vi "Initialise.vi"(8 "error in (no error)":errorcluster, 10 "Message in":refnum<class "InitialiseMessage.lvclass">, 11 "StageSPIM in":refnum<class "StageSPIM.lvclass">) -> (0 "error out":errorcluster, 3 "StageSPIM out":refnum<class "StageSPIM.lvclass">)   [LabVIEW 2012, in "StageSPIM.lvclass"]
doc: "This method is called when an initialise message is received. It mainly initialises the RabbitMQ connectivity. \n\nOverride this method when your component needs special initialisation (e.g. of software or hardware resources). In that case, don't forget to call the parent for proper implementation. If your component owns subcomponents, they count as resources, so you have to initialise them by calling their own initialise functions"
uses:
  StageSPIM.lvclass
  <vilib>/Distrio/Murmex/InitialiseMessage/InitialiseMessage.lvclass
  <vilib>/Distrio/Murmex/Murmex/Murmex.lvclass
  StageSPIM.lvclass/StageSPIM.ctl
panel:
  # "This method is called when the INTIALISE\ntrigger is sent. \n\nOverride this method when your component needs to\nrespond to this trigger. \n\nCall parent for proper implementation"
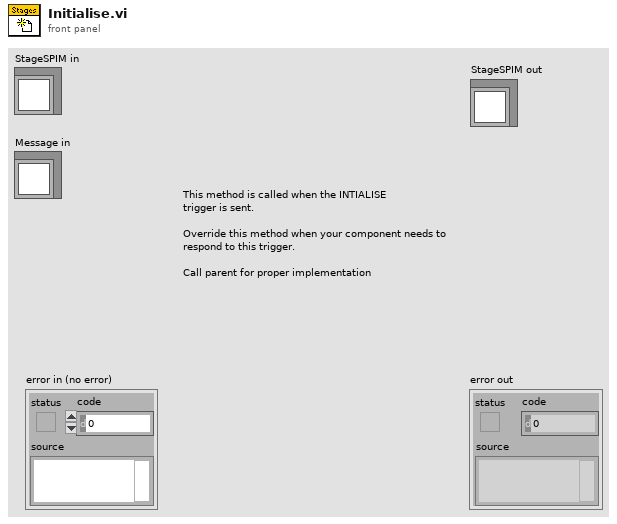
[diagram p1: front panel]
types:
  T1 = cluster{"Register DC":bool, "DaisyChain Search?":bool, "Device ID":i32}[][]
  T2 = cluster{"RON Affected axes":string[], "Reference mode":bool[], "Check FRF?":bool}
  T3 = typedef "StageSPIM.lvclass/port_control.ctl" = i32
  T4 = typedef "StageSPIM.lvclass/baud_rate_control.ctl" = u16
  T5 = typedef "StageSPIM.lvclass/connection_type.ctl" = enum16{"RS232", "RS232 DaisyChain", "USB", "USB_DaisyChain"}
  T6 = cluster{"Register DC":bool, "DaisyChain Search?":bool, "Device ID":i32}
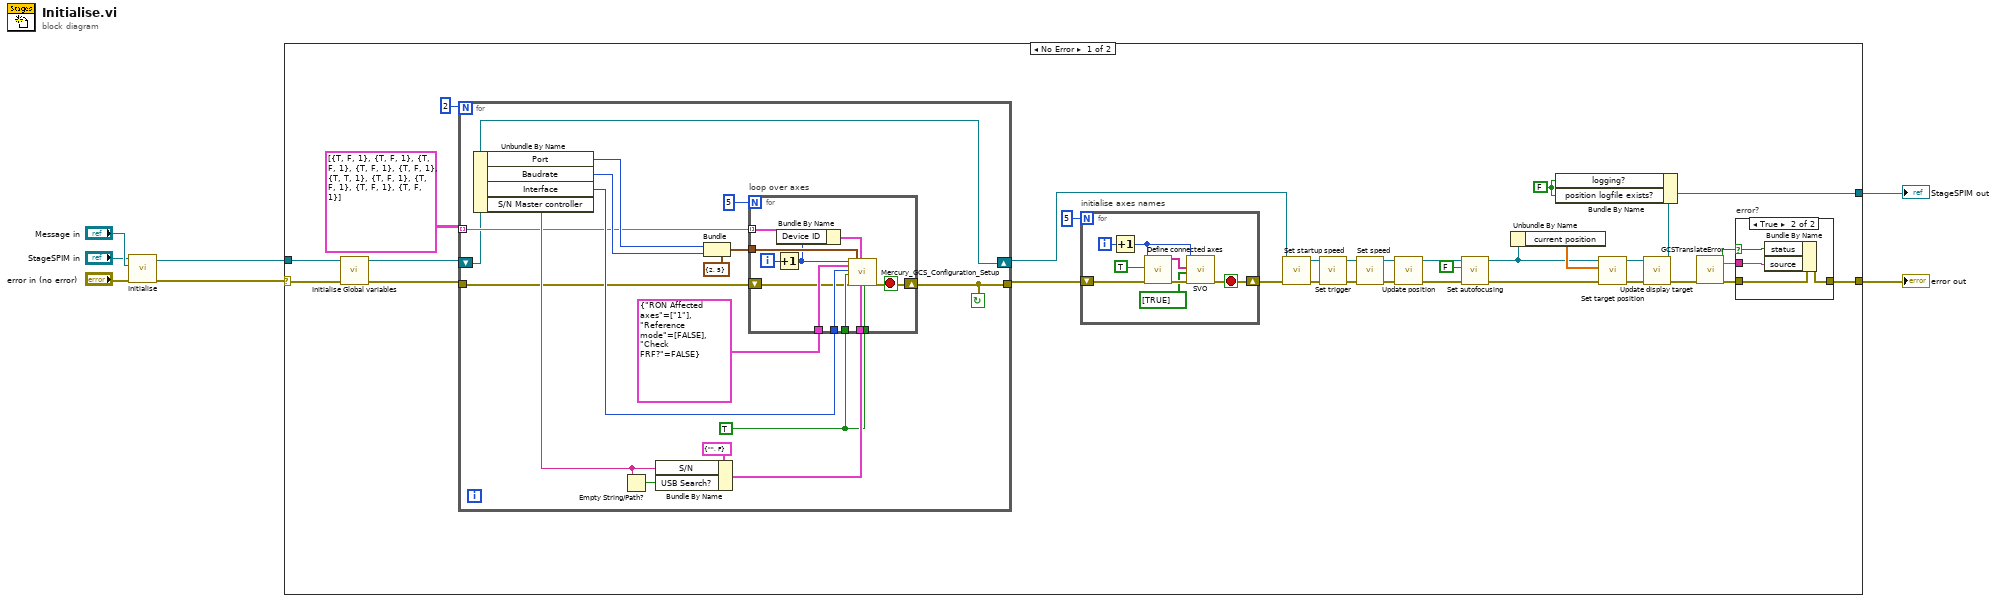
[diagram p0: block diagram]
diagram:
  n1 = call-parent "Initialise.vi"("error in (no error)"="error in (no error)", "Message in"="Message in", "Murmex in"="StageSPIM in") -> ("error out"=w4:errorcluster, "Murmex out"=w3:refnum<class "StageSPIM.lvclass">)  [unwired: 7 in]
  n2 = case shown="No Error" w4 {
    selector: w4 -> [w30 w82]
    tunnel: w3 -> [w28 w81]
    tunnel: [w9 w81] -> w2
    tunnel: [w31 w82] -> w1
    frame No Error {
      w8 = FALSE ("settings.logging?")
      n3 = call-dynamic "Initialise Global variables.vi"("error in (no error)"=w30, "StageSPIM in"=w28) -> ("error out"=w29:errorcluster, "StageSPIM out"=w27:refnum<class "StageSPIM.lvclass">)  [unwired: 8 in]
      n4 = for {
        N: 2 -> [_]
        tunnel: [w41] -> w34
        tunnel: w29 -> [w44]
        tunnel: T1 [[{"Register DC"=TRUE, "DaisyChain Search?"=FALSE, "Device ID"=1}, {"Register DC"=TRUE, "DaisyChain Search?"=FALSE, "Device ID"=1}, {"Register DC"=TRUE, "DaisyChain Search?"=FALSE, "Device ID"=1}, {"Register DC"=TRUE, "DaisyChain Search?"=FALSE, "Device ID"=1}, {"Register DC"=TRUE, "DaisyChain Search?"=FALSE, "Device ID"=1}], [{"Register DC"=TRUE, "DaisyChain Search?"=TRUE, "Device ID"=1}, {"Register DC"=TRUE, "DaisyChain Search?"=FALSE, "Device ID"=1}, {"Register DC"=TRUE, "DaisyChain Search?"=FALSE, "Device ID"=1}, {"Register DC"=TRUE, "DaisyChain Search?"=FALSE, "Device ID"=1}, {"Register DC"=TRUE, "DaisyChain Search?"=FALSE, "Device ID"=1}]] -> [w43] mode=indexing
        shift-right: [w42] -> w17
        shift-left: w27 -> [w42]
        stop <- w41 continue-if-true
        w49 = TRUE ("Switch servo on?")
        n5 = Unbundle By Name(w42) -> ("Port"=w47:T3, "Baudrate"=w46:T4, "Interface"=w45:T5, "S/N Master controller"=w51:string)
        n6 = Empty String/Path?(string/path=w51) -> (empty?=w52:bool)
        n7 = Bundle By Name(cluster=cluster{"S/N":string, "USB Search?":bool} {"S/N"="", "USB Search?"=FALSE} ("USB settings"), "S/N"=w51, "USB Search?"=w52) -> (w50:cluster{"S/N":string, "USB Search?":bool})
        n8 = Bundle(cluster=cluster{"Portnumber":i32, "Baudrate":u16} {"Portnumber"=2, "Baudrate"=5} ("RS232 settings"), "Portnumber"=w47, "Baudrate"=w46) -> (w54:cluster{"Portnumber":i32, "Baudrate":u16})
        n9 = for "loop over axes" {
          N: 5 -> [_]
          tunnel: w43 -> [w60] mode=indexing
          tunnel: w45 -> [w67]
          tunnel: w49 -> [w62]
          tunnel: w54 -> [w66]
          tunnel: T2 {"RON Affected axes"=["1"], "Reference mode"=[FALSE], "Check FRF?"=FALSE} ("RON settings") -> [w65]
          tunnel: w50 -> [w64]
          shift-right: [w63] -> w41
          shift-left: w44 -> [w57]
          tunnel: w49 -> [w61]
          i -> [w56]
          stop <- w63 stop-if-true
          n10 = Increment(x=w56) -> (x+1=w58:i32)
          n11 = Bundle By Name(cluster=w60, "Device ID"=w58) -> (w59:T6)
          n12 = call "Mercury_GCS_Configuration_Setup.vi"("System no."=w58, "RON settings"=w65, "Interface"=w67, "All axes?"=w61, "error in"=w57, "RS232 settings"=w66, "DaisyChain settings"=w59, "USB settings"=w64, "Switch servo on?"=w62) -> ("error out"=w63:errorcluster)  [unwired: 4 in, 6 out]
        }
      }
      n13 = for "initialise axes names" {
        N: 5 -> [_]
        shift-right: [w73] -> w19
        shift-left: w34 -> [w80]
        i -> [w78]
        stop <- w73 stop-if-true
        n14 = Increment(x=w78) -> (x+1=w74:i32)
        n15 = call "Define connected axes.vi"("System no."=w74, "Read from\ncontroller?"=TRUE ("Read from\ncontroller?"), "error in"=w80) -> ("Conn. Axes out"=w75:string[], "error out"=w77:errorcluster)  [unwired: 15 in]
        n16 = call "SVO.vi"("System no."=w74, "Axes to command"=w75, "Servo mode"=bool[] [TRUE], "error in"=w77) -> ("error out"=w73:errorcluster)  [unwired: 15 in]
      }
      n17 = call-dynamic "Set startup speed.vi"("error in (no error)"=w19, "StageSPIM in"=w17) -> ("error out"=w18:errorcluster, "StageSPIM out"=w15:refnum<class "StageSPIM.lvclass">)  [unwired: 8 in]
      n18 = call-dynamic "Set trigger.vi"("error in (no error)"=w18, "StageSPIM in"=w15) -> ("error out"=w16:errorcluster, "StageSPIM out"=w14:refnum<class "StageSPIM.lvclass">)  [unwired: 8 in]
      n19 = call-dynamic "Set speed.vi"("error in (no error)"=w16, "StageSPIM in"=w14) -> ("error out"=w32:errorcluster, "StageSPIM out"=w25:refnum<class "StageSPIM.lvclass">)  [unwired: 8 in]
      n20 = call-dynamic "Update position.vi"("error in (no error)"=w32, "StageSPIM in"=w25) -> ("error out"=w26:errorcluster, "StageSPIM out"=w12:refnum<class "StageSPIM.lvclass">)  [unwired: 8 in]
      n21 = call-dynamic "Set autofocusing.vi"("error in (no error)"=w26, "autofocusing?"=FALSE, "StageSPIM in"=w12) -> ("error out"=w13:errorcluster, "StageSPIM out"=w11:refnum<class "StageSPIM.lvclass">)  [unwired: 7 in]
      n22 = Unbundle By Name(w11) -> ("current position"=w22:dbl[])
      n23 = call-dynamic "Set target position.vi"("error in (no error)"=w13, "target position"=w22, "StageSPIM in"=w11) -> ("error out"=w24:errorcluster, "StageSPIM out"=w21:refnum<class "StageSPIM.lvclass">)  [unwired: 7 in]
      n24 = call-dynamic "Update display target.vi"("error in (no error)"=w24, "StageSPIM in"=w21) -> ("error out"=w23:errorcluster, "StageSPIM out"=w20:refnum<class "StageSPIM.lvclass">)  [unwired: 8 in]
      n25 = Bundle By Name(cluster=w20, "logging?"=w8, "position logfile exists?"=w8) -> (w9:refnum<class "StageSPIM.lvclass">)
      n26 = call "GCSTranslateError.vi"("error in"=w23) -> ("GCS Error?"=w39:bool, "Error Description"=w37:string, "error out"=w38:errorcluster)  [unwired: 16 in]
      n27 = case "error?" shown="True" w39 {
        selector: w39 -> [_ w71]
        tunnel: w38 -> [w68 w72]
        tunnel: w37 -> [_ w70]
        tunnel: [w68 w69] -> w31
        frame False {
        }
        frame True {
          n28 = Bundle By Name(cluster=w72, "status"=w71, "source"=w70) -> (w69:errorcluster)
        }
      }
    }
    frame Error {
    }
  }
  "error out" <- w1
  "StageSPIM out" <- w2
